vi "GetGravityfromQuaternion.vi"(11 "qa":T2) -> (3 "Gravity (out)":T1)   [LabVIEW 2015]
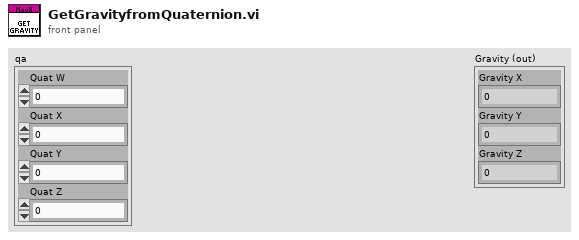
[diagram p1: front panel]
types:
  T1 = cluster{"Gravity X":dbl, "Gravity Y":dbl, "Gravity Z":dbl}
  T2 = cluster{"Quat W":dbl, "Quat X":dbl, "Quat Y":dbl, "Quat Z":dbl}
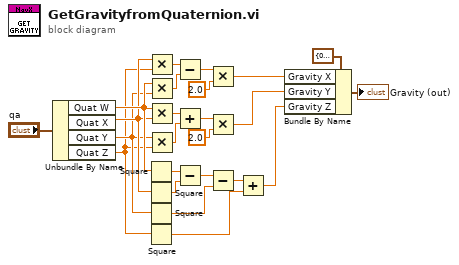
[diagram p0: block diagram]
diagram:
  n1 = Unbundle By Name("qa") -> ("Quat W"=w5:dbl, "Quat X"=w4:dbl, "Quat Y"=w3:dbl, "Quat Z"=w2:dbl)
  n2 = Square(x=w5) -> (x^2=w9:dbl)
  n3 = Square(x=w4) -> (x^2=w8:dbl)
  n4 = Square(x=w3) -> (x^2=w7:dbl)
  n5 = Square(x=w2) -> (x^2=w6:dbl)
  n6 = Multiply(x=w4, y=w2) -> (x*y=w23:dbl)
  n7 = Multiply(x=w5, y=w3) -> (x*y=w22:dbl)
  n8 = Multiply(x=w5, y=w4) -> (x*y=w13:dbl)
  n9 = Multiply(x=w3, y=w2) -> (x*y=w14:dbl)
  n10 = Subtract(x=w23, y=w22) -> (x-y=w21:dbl)
  n11 = Add(x=w13, y=w14) -> (x+y=w15:dbl)
  n12 = Subtract(x=w9, y=w8) -> (x-y=w11:dbl)
  n13 = Multiply(x=w21, y=2.0) -> (x*y=w17:dbl)
  n14 = Multiply(x=w15, y=2.0) -> (x*y=w12:dbl)
  n15 = Subtract(x=w11, y=w7) -> (x-y=w10:dbl)
  n16 = Add(x=w10, y=w6) -> (x+y=w1:dbl)
  n17 = Bundle By Name(cluster=T1 {"Gravity X"=0.0, "Gravity Y"=0.0, "Gravity Z"=0.0} ("Gravity (out)"), "Gravity X"=w17, "Gravity Y"=w12, "Gravity Z"=w1) -> (→"Gravity (out)":T1)
